vi "Teleop.vi"(10 "Match Info":T1={"Autonomous Elapsed Seconds"=0.0, "TeleOp Elapsed Seconds"=7.961, "Disabled Elapsed Seconds"=0.0, "Visited Autonomous"=FALSE, "Visited TeleOp"=TRUE, "Visited Disabled"=FALSE, "Autonomous Settings"={"Autonomous Style"=enum."Independent", "VI Refnum"=refnum}}, 11 "Call Context":T2=enum."Execute") -> ()   [LabVIEW 2016]
doc: "This VI is called for each TeleOp packet received from the DS where the robot is not disabled. It is often used to read from the joysticks and update I/O or to update setpoints for timed control loops. It should complete and return within 20 milliseconds or it may miss DS packets."
uses:
  <vilib>/Rock Robotics/WPI/DriverStation/WPI_DriverStationDerivedRobotMode.ctl
  <vilib>/Rock Robotics/WPI/DriverStation/WPI_DriverStationMatch Info.ctl
panel:
  out "Neither?":bool
  out "Gears?":bool
  out "Balls?":bool
  in  "Neither":bool
  in  "Gears":bool
  in  "Balls":bool
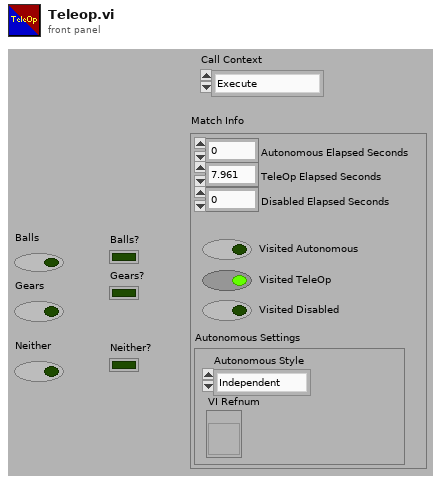
[diagram p1: front panel]
types:
  T1 = typedef "WPI_DriverStationMatch Info.ctl" = cluster{"Autonomous Elapsed Seconds":dbl, "TeleOp Elapsed Seconds":dbl, "Disabled Elapsed Seconds":dbl, "Visited Autonomous":bool, "Visited TeleOp":bool, "Visited Disabled":bool, "Autonomous Settings":cluster{"Autonomous Style":enum16{"Iterative", "Independent"}, "VI Refnum":refnum<vi>}}
  T2 = typedef "WPI_DriverStationDerivedRobotMode.ctl" = enum16{"Init", "Execute", "Stop"}
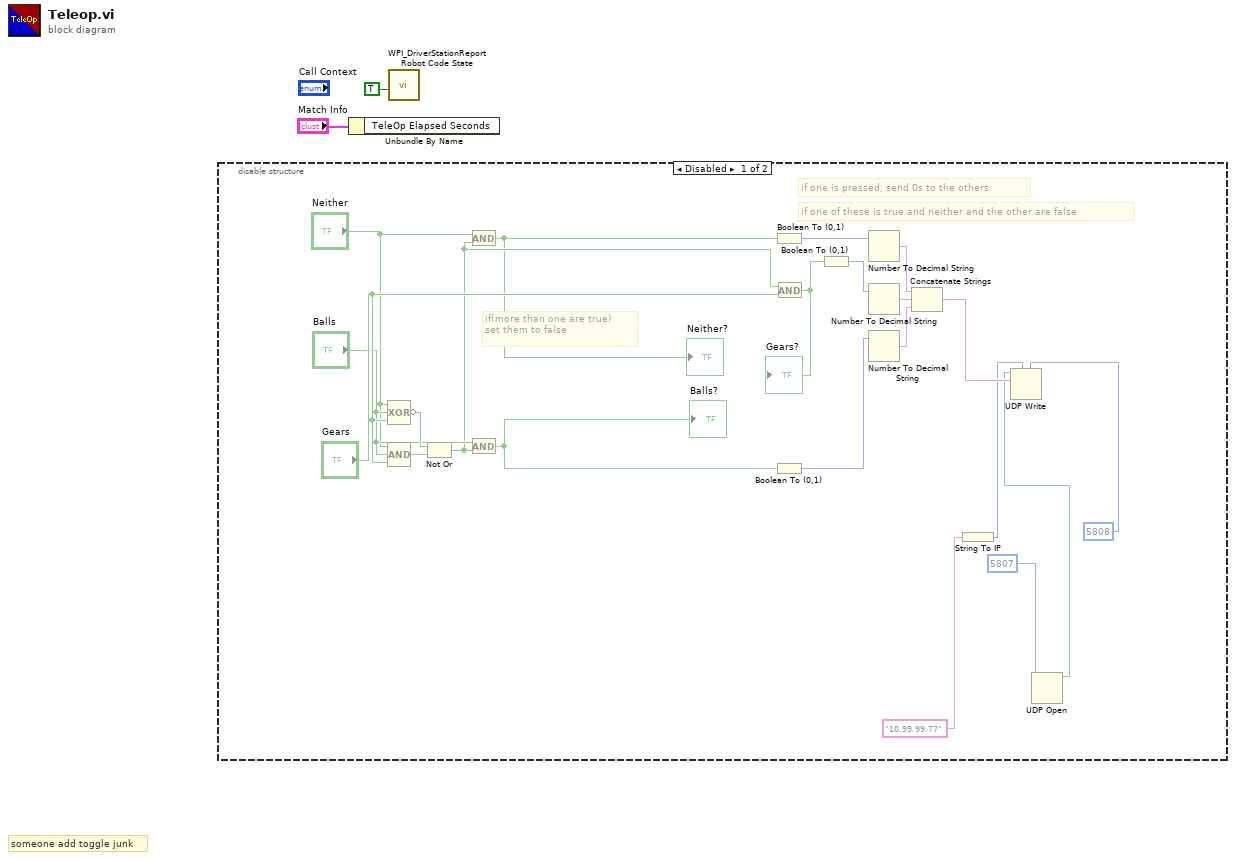
[diagram p0: block diagram]
diagram:
  # "someone add toggle junk"
  n1 = disable-structure shown="Disabled" {
    frame Disabled {
      # "if one is pressed, send 0s to the others"
      # "if one of these is true and neither and the other are false"
      # "if(more than one are true)\nset them to false"
      n2 = Compound Arithmetic op=XOR("Neither", "Balls", "Gears") -> (invert w18:bool)
      n3 = Compound Arithmetic op=AND("Neither", "Balls", "Gears") -> (w14:bool)
      n4 = Not Or(1:w14, 2:w18) -> (0:w13:bool)
      n5 = And(x="Neither", y=w13) -> (x .and. y?=w12:bool)
      "Neither?" <- w12
      n6 = And(x="Balls", y=w13) -> (x .and. y?=w8:bool)
      "Balls?" <- w8
      n7 = Boolean To (0,1)(Boolean=w12) -> (0, 1=w11:i16)
      n8 = Boolean To (0,1)(Boolean=w8) -> (0, 1=w7:i16)
      n9 = And(x=w13, y="Gears") -> (x .and. y?=w9:bool)
      "Gears?" <- w9
      n10 = Boolean To (0,1)(Boolean=w9) -> (0, 1=w10:i16)
      n11 = Number To Decimal String(number=w11) -> (decimal integer string=w21:string)  [unwired: 1 in]
      n12 = Number To Decimal String(number=w10) -> (decimal integer string=w19:string)  [unwired: 1 in]
      n13 = Number To Decimal String(number=w7) -> (decimal integer string=w20:string)  [unwired: 1 in]
      n14 = Concatenate Strings(w21, w19, w20) -> (w6:string)
      n15 = String To IP(1:"10.99.99.77" ("name")) -> (0:w5:u32)
      n16 = UDP Open(11:u16 5807 ("port")) -> (port=w3:refnum<k16>)  [unwired: 4 in, 2 out]
      n17 = UDP Write(address=w5, port or service name=u16 5808, connection ID=w3, data in=w6) -> ()  [unwired: 2 in, 2 out]
    }
    frame Enabled {
    }
  }
  n18 = Unbundle By Name("Match Info") -> ()  [unwired: 1 out]
  n19 = call <vilib>:"WPI_DriverStationReport Robot Code State.vi"("TeleOp"=TRUE ("Autonomous")) -> ()  [unwired: 10 in, 1 out]
